vi "TriangleArea.vi"() -> ()   [LabVIEW 2024]
panel:
  in  "stop":bool
  in  "Height(cm)":dbl
  in  "Base(cm)":dbl
  out "Area":dbl
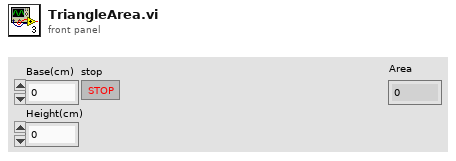
[diagram p1: front panel]
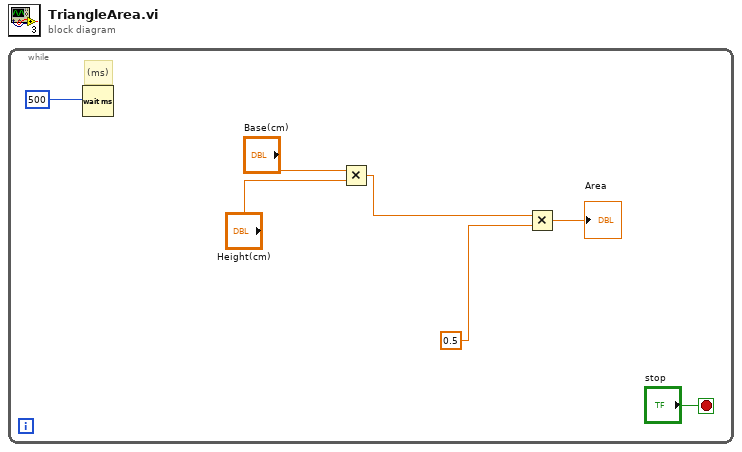
[diagram p0: block diagram]
diagram:
  n1 = while {
    stop <- "stop" stop-if-true
    # "(ms)"
    n2 = Wait (ms)(milliseconds to wait=u32 500 ("millisecond timer value")) -> ()  [unwired: 1 out]
    n3 = Multiply(x="Base(cm)", y="Height(cm)") -> (x*y=w3:dbl)
    n4 = Multiply(x=w3, y=0.5) -> (x*y=→"Area":dbl)
  }
